vi "Icai 105 - Simultry_9_express.vi"() -> ()   [LabVIEW 2010]
uses:
  <vilib>/Utility/error.llb/DialogType.ctl
  <vilib>/DAQmx/write.llb/DAQmx Write (Analog DBL 1Chan 1Samp).vi
  <vilib>/DAQmx/write.llb/DAQmx Write (Digital 1D Bool 1Chan 1Samp).vi
  <vilib>/DAQmx/write.llb/DAQmx Write (Analog Wfm 1Chan NSamp).vi
  <vilib>/DAQmx/create/channels.llb/DAQmx Create Channel (AO-Voltage-Basic).vi
  <vilib>/daqmx/miscellaneous.llb/DAQmx Fill In Error Info.vi
  <vilib>/Waveform/WDTOps.llb/WDT Append Waveforms DBL.vi
  <vilib>/measure/matone.llb/Extract Single Tone Information 1 Chan.vi
  <vilib>/DAQmx/create/channels.llb/DAQmx Create Channel (DO-Digital Output).vi
  <vilib>/DAQmx/configure/timing.llb/DAQmx Timing (Sample Clock).vi
  <vilib>/measure/NI_MABase.lvlib
  <vilib>/measure/NI_MAPro.lvlib
  Program Files/National Instruments/LabVIEW 2010/resource/objmgr/daqmx.rc
panel:
  in  "rate":dbl=10000000.0
  out "detected frequency 2":dbl format="%.6p"
  out "SampClk.Timebase.Rate":dbl format="%^#_10g"
  in  "Freq Scale Factor":dbl=1.6405228 format="%#_12g"
  out "detected frequency":dbl format="%.6p"
  out "signal out":waveform(dbl)(graph)
  in  "lines":tag="Dev1/port0/line3"
  in  "Rising Logic Output Chan":tag="Dev1/ao2"
  in  "Mod Duration ms":i32=300
  in  "Samples (1Ms/s)":i32=700000
  out "min value":dbl
  in  "Falling Logic Output Chan":tag="Dev1/ao1"
  in  "FM Waveform Channel":tag="Dev1/ao3"
  out "error out":errorcluster caption="error out (DAQ)"
  out "Mod":dbl=118572.0
  out "Numeric 2":dbl=3900000.0 format="%#_7g"
  out "Numeric":dbl=3900000.0 format="%#_7g"
  in  "Pre-Trig Samples":ext=100.0 format="%.2f"
  out "?":dbl=579698.7113293351 format="%#_6f"
  in  "Fs":dbl=1000000.0
  out "#s":dbl=39524.02451426849
  in  "Time int":i32=30000
  in  "Sensitivity":u16(ring)=14 items=["2 nV/fA", "5 nV/fA", "10 nV/fA", "20 nV/fA", "50 nV/fA", "100 nV/fA", "200 nV/fA", "500 nV/fA", "1 uV/pA", "2 uV/pA", "5 uV/pA", "10 uV/pA", "20 uV/pA", "50 uV/pA", "100 uV/pA", "200 uV/pA", "500 uV/pA", "1 mV/nA", "2 mV/nA", "5 mV/nA", "10 mV/nA", "20 mV/nA", "50 mV/nA", "100 mV/nA", "200 mV/nA", "500 mV/nA", "1 V/uA"]
  in  "Detection Bandwidth":u16(ring)=7 items=["10 us/ 25 kHz", "30 us /8.33 kHz", "100 us/ 2.50 kHz", "300 us/ 833 Hz", "1 ms /250 Hz", "3 ms /83.3 Hz", "10 ms/ 25 Hz", "30 ms/ 8.33 Hz", "100 ms/ 2.50 Hz", "300 ms/ 0.833 Hz ", "1 s/ 0.250 Hz", "3 s/ 0.0833 Hz", "10 s/0.025 Hz"]
  in  "SR 830 GPIB Address":i32=8
  in  "Freq 2":dbl=2448.0 format="%_7g"
  out "Iterat #":dbl=10.0
  in  "Iteration":dbl=17.0
  in  "stop 2":bool
  in  "pulse":bool=TRUE
  in  "Start":ext=0.05
  out "?":waveform(dbl)[](graph)
  in  "amplitude 2":dbl=0.25 format="%0.2p"
  in  "?":T1(ring)=enum."Triangle Wave"
  in  "phase 2":dbl format="%.2p"
  in  "Offset 2":dbl=-0.0 format="%#_6p"
  in  "frequency 4":dbl=100.0 format="%0.2p"
  in  "sampling info 4":cluster{"Fs":dbl, "#s":dbl}={"Fs"=1000000.0, "#s"=2500.0} {"Fs" format="%.2p"}
  in  "?":T1(ring)=enum."Triangle Wave"
  in  "offset 4":dbl=-1.0 format="%0.2p"
  in  "phase 4":dbl=90.0 format="%.2p"
  in  "amplitude 4":dbl=1.0 format="%0.2p"
  in  "frequency 1":dbl=100.0 format="%0.2p"
  in  "amplitude 1":dbl=1.0 format="%0.2p"
  in  "sampling info 1":cluster{"Fs":dbl, "#s":dbl}={"Fs"=1000000.0, "#s"=2500.0} {"Fs" format="%.2p"}
  in  "?":T1(ring)=enum."Triangle Wave"
  in  "phase 1":dbl=-90.0 format="%.2p"
  in  "Offset 1":dbl format="%#_6p"
  in  "iterat":dbl
  out "CW":dbl=123571.0
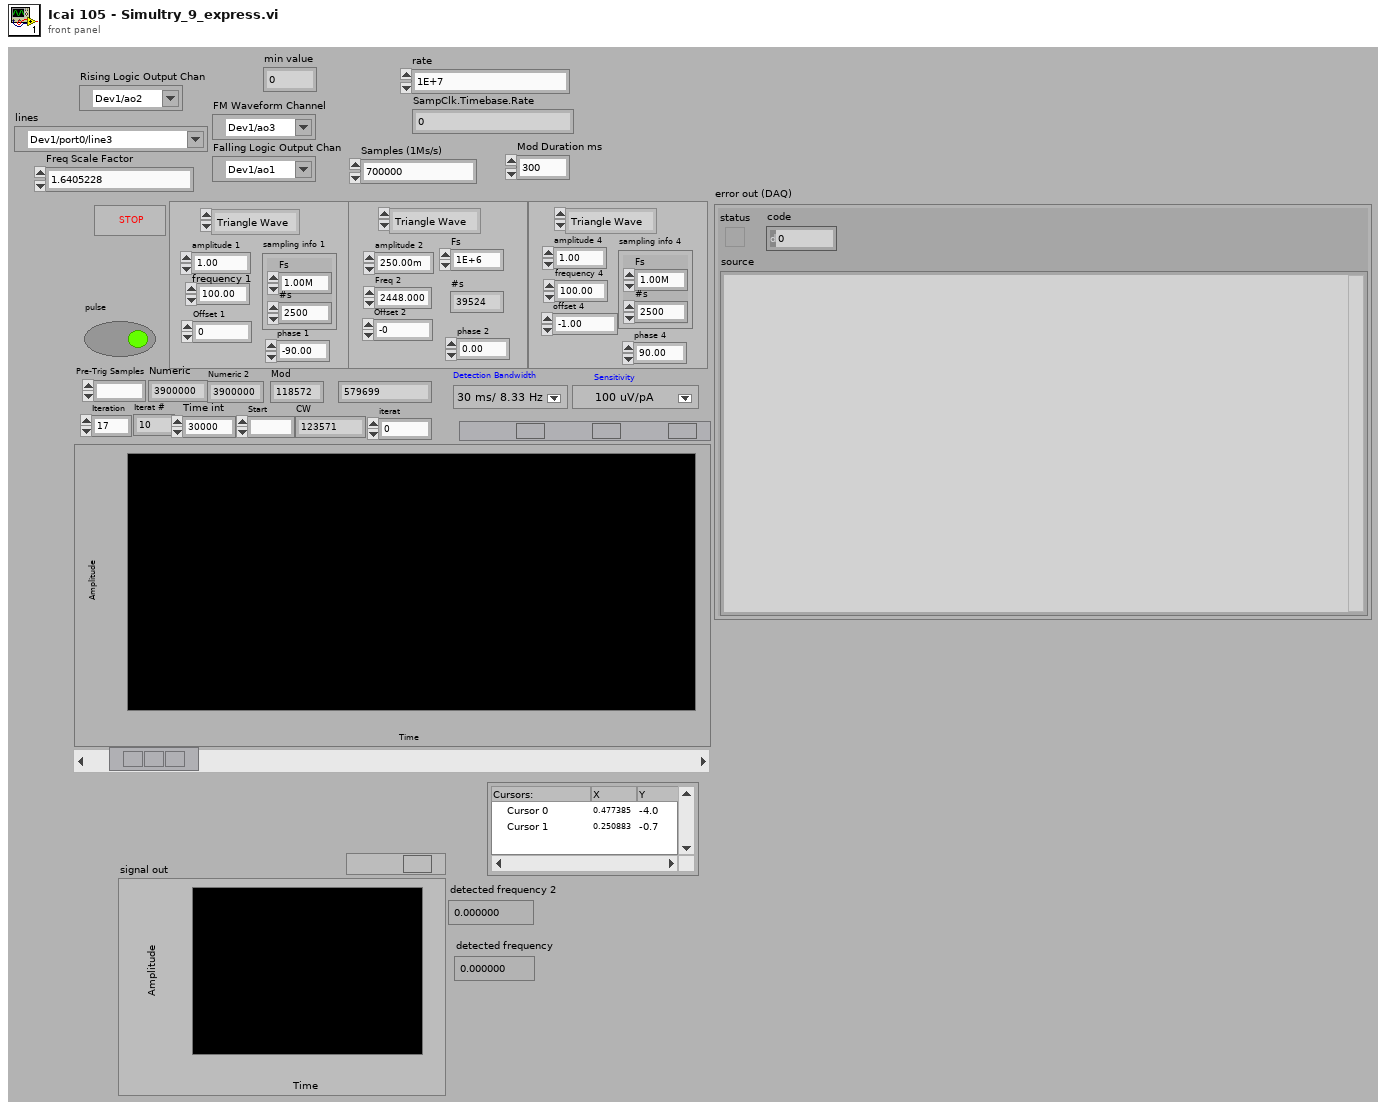
[diagram p1: front panel]
types:
  T1 = enum16{"Sine Wave", "Triangle Wave", "Square Wave", "Sawtooth Wave"}
  T2 = typedef "DialogType.ctl" = u16
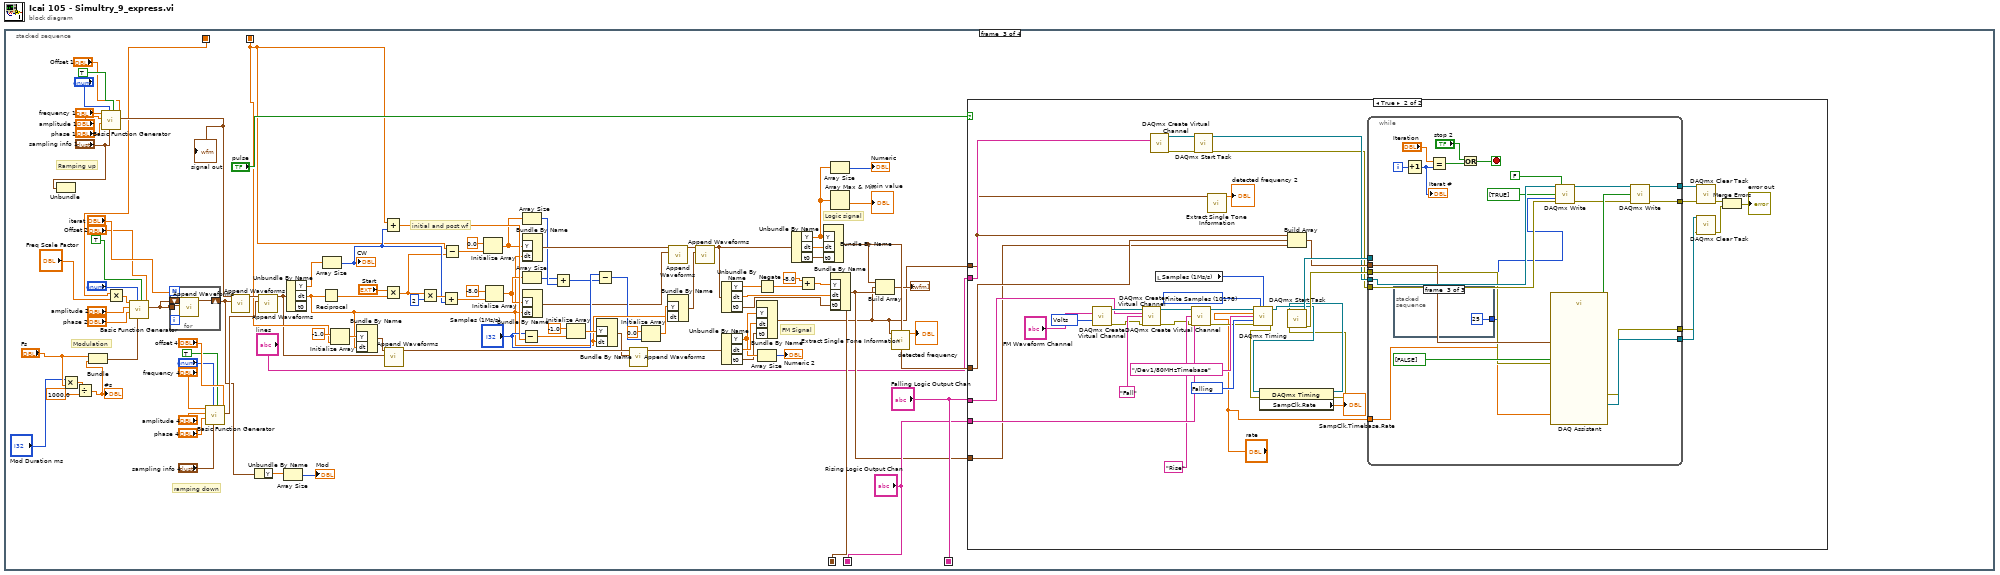
[diagram p0: block diagram]
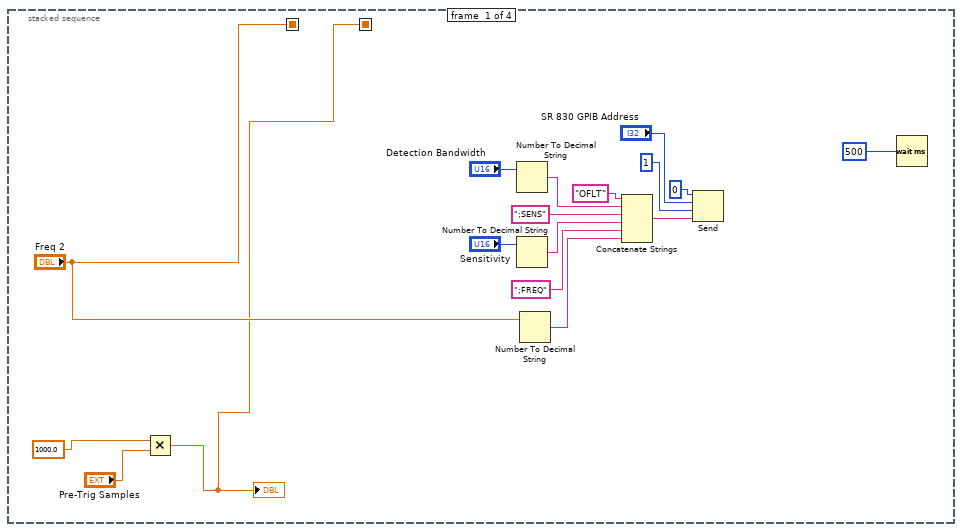
[diagram p2: hidden frame]
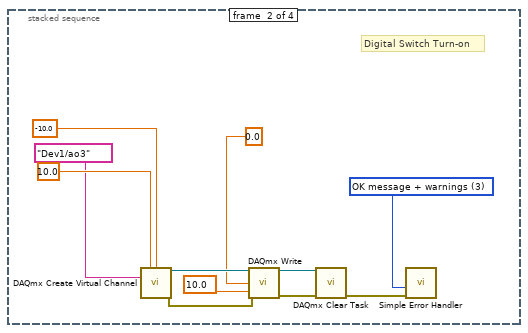
[diagram p3: hidden frame]
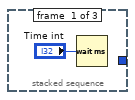
[diagram p5: hidden frame]
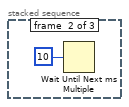
[diagram p6: hidden frame]
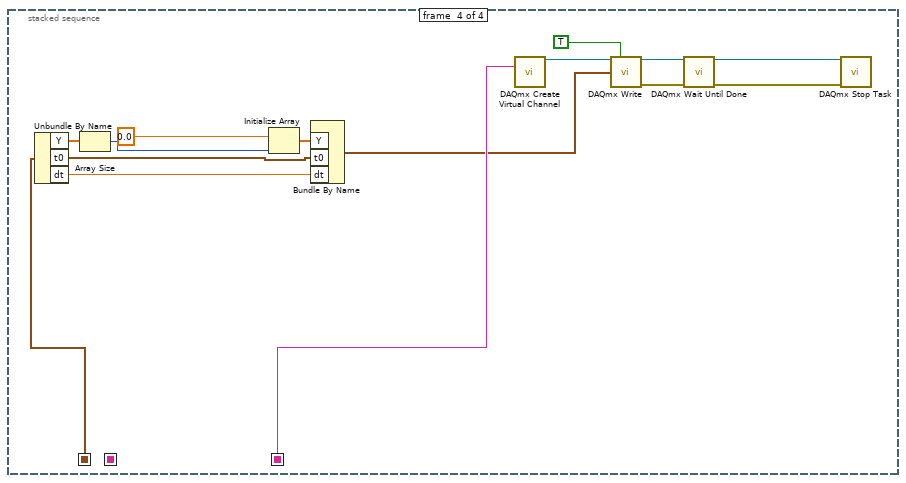
[diagram p7: hidden frame]
diagram:
  n1 = stacked-sequence {
    seq-local: ["Freq 2" _ _ _] -> [_ _ w31 _]
    seq-local: [w1 _ _ _] -> [_ _ w68 _]
    seq-local: [_ _ "Falling Logic Output Chan" _] -> [_ _ _ w196]
    seq-local: [_ _ "Rising Logic Output Chan" _] -> [_ _ _ _]
    seq-local: [_ _ w48 _] -> [_ _ _ w204]
    frame #0 {
      n2 = Multiply(x=1000.0 ("Fs 2"), y="Pre-Trig Samples") -> (x*y=w1:ext)
      "?" <- w1
      n3 = Number To Decimal String(number="Detection Bandwidth") -> (decimal integer string=w16:string)  [unwired: 1 out]
      n4 = Number To Decimal String(number="Sensitivity") -> (decimal integer string=w14:string)  [unwired: 1 out]
      n5 = Number To Decimal String(number="Freq 2") -> (decimal integer string=w5:string)  [unwired: 1 out]
      n6 = Concatenate Strings("OFLT", w16, ";SENS", w14, ";FREQ" ("string"), w5) -> (w13:string)
      n7 = Send(0:0 ("bus"), 2:"SR 830 GPIB Address", 3:i16 1 ("mode"), 5:w13) -> ()  [unwired: 1 in, 3 out]
      n8 = Wait (ms)(milliseconds to wait=500) -> ()  [unwired: 1 out]
    }
    frame #1 {
      w21 = T2 3 items=["no dialog", "OK message", "continue or stop message", "OK message + warnings", "continue/stop + warnings"] ("type of dialog (OK msg:1)")
      # "Digital Switch Turn-on"
      n9 = call-poly <vilib>:"DAQmx Create Virtual Channel.vi"("maximum value"=10.0 ("Maximum Value"), "minimum value"=-10.0 ("Minimum Value"), "physical channels"=tag "Dev1/ao3" ("Physical Channel")) -> ("task out"=w24:refnum<k21>, "error out"=w25:errorcluster)  [unwired: 6 in, 5 out]
      n10 = call-poly <vilib>:"DAQmx Write.vi"("task/channels in"=w24, "data"=0.0 ("Voltage Output"), "timeout"=10.0, "error in"=w25) -> ("task out"=w19:refnum<k21>, "error out"=w20:errorcluster)  [unwired: 1 in, 9 out]
      n11 = call <vilib>:"DAQmx Clear Task.vi"("task in"=w19, "error in"=w20) -> ("error out"=w18:errorcluster)  [unwired: 13 out]
      n12 = call <vilib>:"Simple Error Handler.vi"("type of dialog (OK msg:1)"=w21, "error in (no error)"=w18) -> ()  [unwired: 8 out]
    }
    frame #2 {
      # "initial and post wf"
      # "FM Signal"
      # "Logic signal"
      # "Ramping up"
      # "ramping down"
      # "Modulation"
      n13 = Unbundle("sampling info 1") -> ()  [unwired: 2 out]
      n14 = Multiply(x="Mod Duration ms", y="Fs") -> (x*y=w38:dbl)
      n15 = Divide(x=w38, y=1000.0) -> (x/y=w36:dbl)
      "#s" <- w36
      n16 = Bundle("Fs"="Fs", w36) -> (w72:cluster{"Fs":dbl, dbl})  [unwired: 1 out]
      n17 = call <vilib>:"Basic Function Generator.vi"("offset"="Offset 1", "reset signal"=TRUE, "sampling info"="sampling info 1", "signal type"="?", "phase"="phase 1", "amplitude"="amplitude 1", "frequency"="frequency 1") -> ("signal out"=w106:waveform(dbl))  [unwired: 2 in, 2 out]
      "signal out" <- w106
      n18 = Multiply(x=w31, y="Freq Scale Factor") -> (x*y=w30:dbl)
      n19 = call <vilib>:"Basic Function Generator.vi"("offset"="Offset 2", "reset signal"=TRUE, "sampling info"=w72, "signal type"="?", "phase"="phase 2", "amplitude"="amplitude 2", "frequency"=w30) -> ("signal out"=w34:waveform(dbl))  [unwired: 2 in, 2 out]
      n20 = for {
        N: "iterat" -> [_]
        shift-right: [w194] -> w61
        shift-left: w34 -> [w192]
        tunnel: w34 -> [w193]
        n21 = call-poly <vilib>:"Append Waveforms.vi"("waveform B"=w193, "waveform A"=w192) -> ("waveform out"=w194:waveform(dbl))  [unwired: 1 in, 8 out]
      }
      n22 = call <vilib>:"Basic Function Generator.vi"("offset"="offset 4", "reset signal"=TRUE, "sampling info"="sampling info 4", "signal type"="?", "phase"="phase 4", "amplitude"="amplitude 4", "frequency"="frequency 4") -> ("signal out"=w111:waveform(dbl))  [unwired: 2 in, 2 out]
      n23 = call-poly <vilib>:"Append Waveforms.vi"("waveform B"=w61, "waveform A"=w106) -> ("waveform out"=w105:waveform(dbl))  [unwired: 1 in, 8 out]
      n24 = Unbundle By Name(w61) -> ("Y"=w62:dbl[])
      n25 = call-poly <vilib>:"Append Waveforms.vi"("waveform B"=w111, "waveform A"=w105) -> ("waveform out"=w44:waveform(dbl))  [unwired: 1 in, 8 out]
      n26 = Array Size(array=w62) -> (size(s)=→"Mod":i32)
      n27 = Unbundle By Name(w44) -> ("Y"=w107:dbl[], "dt"=w67:dbl)  [unwired: 1 out]
      n28 = Reciprocal(x=w67) -> (1/x=w69:dbl)
      n29 = Array Size(array=w107) -> (size(s)=w89:i32)
      "CW" <- w89
      n30 = Initialize Array(-1.0 ("DC level"), w68) -> (w96:dbl[])
      n31 = Bundle By Name("Y"=w96, "dt"=w67) -> (w109:waveform(dbl))  [unwired: 1 out]
      n32 = Add(x=w68, y=w89) -> (x+y=w94:ext)
      n33 = Multiply(x="Start", y=w69) -> (x*y=w82:ext)
      n34 = call-poly <vilib>:"Append Waveforms.vi"("waveform B"=w44, "waveform A"=w109) -> ("waveform out"=w110:waveform(dbl))  [unwired: 1 in, 8 out]
      n35 = Multiply(x=w82, y=2) -> (x*y=w90:ext)
      n36 = Add(x=w90, y=w89) -> (x+y=w71:ext)
      n37 = Subtract(x=w68, y=w82) -> (x-y=w83:ext)
      n38 = Initialize Array(0.0 ("Trigger down"), w83) -> (w81:dbl[])
      n39 = Initialize Array(-8.0 ("Trigger up"), w71) -> (w80:dbl[])
      n40 = Subtract(x="Samples (1Ms/s)", y=w94) -> (x-y=w93:ext)
      n41 = Bundle By Name("Y"=w81, "dt"=w67) -> (w85:waveform(dbl))  [unwired: 1 out]
      n42 = Bundle By Name("Y"=w80, "dt"=w67) -> (w42:waveform(dbl))  [unwired: 1 out]
      n43 = Array Size(array=w81) -> (size(s)=w79:i32)
      n44 = Array Size(array=w80) -> (size(s)=w78:i32)
      n45 = Add(x=w78, y=w79) -> (x+y=w77:i32)
      n46 = Initialize Array(-1.0 ("DC level"), w93) -> (w92:dbl[])
      n47 = Subtract(x="Samples (1Ms/s)", y=w77) -> (x-y=w43:i32)
      n48 = Bundle By Name("Y"=w92, "dt"=w67) -> (w91:waveform(dbl))  [unwired: 1 out]
      n49 = call-poly <vilib>:"Append Waveforms.vi"("waveform B"=w91, "waveform A"=w110) -> ("waveform out"=w99:waveform(dbl))  [unwired: 1 in, 8 out]
      n50 = Initialize Array(0.0 ("Trigger down"), w43) -> (w86:dbl[])
      n51 = Bundle By Name("Y"=w86, "dt"=w67) -> (w84:waveform(dbl))  [unwired: 1 out]
      n52 = call-poly <vilib>:"Append Waveforms.vi"("waveform B"=w42, "waveform A"=w85) -> ("waveform out"=w102:waveform(dbl))  [unwired: 1 in, 8 out]
      n53 = call-poly <vilib>:"Append Waveforms.vi"("waveform B"=w84, "waveform A"=w102) -> ("waveform out"=w59:waveform(dbl))  [unwired: 1 in, 8 out]
      n54 = Unbundle By Name(w59) -> ("Y"=w58:dbl[], "dt"=w53:dbl, "t0"=w54:timestamp)
      n55 = Unbundle By Name(w99) -> ("Y"=w64:dbl[], "dt"=w98:dbl, "t0"=w41:timestamp)
      n56 = Bundle By Name("Y"=w64, "dt"=w98, "t0"=w41) -> (w32:waveform(dbl))  [unwired: 1 out]
      n57 = Negate(x=w58) -> (-x=w56:dbl[])
      n58 = Array Size(array=w64) -> (size(s)=→"Numeric 2":i32)
      n59 = Unbundle By Name(w59) -> ("Y"=w60:dbl[], "dt"=w100:dbl, "t0"=w55:timestamp)
      n60 = Add(x=-8.0, y=w56) -> (x+y=w52:dbl[])
      n61 = Bundle By Name("Y"=w60, "dt"=w100, "t0"=w55) -> (w47:waveform(dbl))  [unwired: 1 out]
      n62 = Bundle By Name("Y"=w52, "dt"=w53, "t0"=w54) -> (w48:waveform(dbl))  [unwired: 1 out]
      n63 = Array Size(array=w60) -> (size(s)=→"Numeric":i32)
      n64 = Array Max & Min(array=w60) -> (min value=→"min value":dbl)  [unwired: 3 out]
      n65 = Build Array(w47, w32, w48) -> (→"?":waveform(dbl)[])
      n66 = call-poly <vilib>:"Extract Single Tone Information.vi"("time signal in"=w32) -> ("detected frequency"=→"detected frequency":dbl)  [unwired: 5 in, 5 out]
      n67 = case shown="True" "pulse" {
        tunnel: w32 -> [_ w130]
        tunnel: w47 -> [_ w152]
        tunnel: w48 -> [_ w132]
        tunnel: "Falling Logic Output Chan" -> [_ w165]
        tunnel: "Rising Logic Output Chan" -> [_ w162]
        tunnel: "lines" -> [_ w149]
        frame False {
        }
        frame True {
          w138 = 10348 items=["Volts"=10348, "From Custom Scale"=10065] ("units")
          w157 = 10178 items=["Finite Samples"=10178, "Continuous Samples"=10123, "Hardware Timed Single Point"=12522] ("sample mode")
          w158 = 10171 items=["Rising"=10280, "Falling"=10171] ("active edge")
          n68 = call-poly <vilib>:"DAQmx Create Virtual Channel.vi"("physical channels"="FM Waveform Channel", "units"=w138) -> ("task out"=w166:refnum<k21>, "error out"=w154:errorcluster)  [unwired: 12 in]
          n69 = call-poly <vilib>:"DAQmx Create Virtual Channel.vi"("task in"=w166, "physical channels"=w165, "name to assign"="Fall", "error in"=w154) -> ("task out"=w163:refnum<k21>, "error out"=w155:errorcluster)  [unwired: 10 in]
          n70 = call-poly <vilib>:"DAQmx Create Virtual Channel.vi"("lines"=w149) -> ("task out"=w145:refnum<k21>, "error out"=w139:errorcluster)  [unwired: 13 in]
          n71 = local read "Samples (1Ms/s)"() -> (w146:i32)
          n72 = call-poly <vilib>:"DAQmx Create Virtual Channel.vi"("task in"=w163, "physical channels"=w162, "name to assign"="Rise", "error in"=w155) -> ("task out"=w160:refnum<k21>, "error out"=w156:errorcluster)  [unwired: 10 in]
          n73 = call <vilib>:"DAQmx Start Task.vi"("task/channels in"=w145, "error in"=w139) -> ("task out"=w148:refnum<k21>, "error out"=w147:errorcluster)  [unwired: 12 in]
          n74 = call-poly <vilib>:"Extract Single Tone Information.vi"("time signal in"=w130) -> ("detected frequency"=→"detected frequency 2":dbl)  [unwired: 5 in, 5 out]
          n75 = call-poly <vilib>:"DAQmx Timing.vi"("task/channels in"=w160, "sample mode"=w157, "samples per channel"=w146, "rate"="rate", "source"=tag "/Dev1/80MHzTimebase", "active edge"=w158, "error in"=w156) -> ("task out"=w137:refnum<k21>, "error out"=w134:errorcluster)  [unwired: 7 in]
          n76 = property class="DAQmx Timing"(reference=w137, error in=w134) -> (reference out=w136:refnum<k21>, error out=w135:errorcluster, "SampClk.Rate"=→"SampClk.Timebase.Rate":dbl)
          n77 = call <vilib>:"DAQmx Start Task.vi"("task/channels in"=w136, "error in"=w135) -> ("task out"=w153:refnum<k21>, "error out"=w150:errorcluster)  [unwired: 12 in]
          n78 = Build Array(w130, w152, w132) -> (w151:waveform(dbl)[])
          n79 = while {
            tunnel: w153 -> [_]
            tunnel: w151 -> [w173]
            tunnel: w150 -> [w172]
            tunnel: w148 -> [w182]
            tunnel: w147 -> [w180]
            tunnel: [w175] -> w143
            tunnel: [w174] -> w144
            tunnel: [w171] -> w129
            tunnel: [w170] -> w128
            tunnel: "rate" -> [w169]
            i -> [w185]
            stop <- w186 stop-if-true
            n80 = stacked-sequence {
              tunnel: [_ _ 25 ("timeout (s)")] -> w168
              frame #0 {
                n81 = Wait (ms)(milliseconds to wait="Time int") -> ()  [unwired: 1 out]
              }
              frame #1 {
                n82 = Wait Until Next ms Multiple(millisecond multiple=u32 10) -> ()  [unwired: 1 out]
              }
              frame #2 {
              }
            }
            n83 = Increment(x=w185) -> (x+1=w183:i32)
            "Iterat #" <- w183
            n84 = Equal?(x="Iteration", y=w183) -> (x = y?=w188:bool)
            n85 = Or(x="stop 2", y=w188) -> (x .or. y?=w186:bool)
            n86 = call "DAQ Assistant"("data"=w173, "rate"=w169, "error in"=w172) -> ("task out"=w171:refnum<k21>, "error out"=w170:errorcluster)  [unwired: 15 in]
            n87 = call-poly <vilib>:"DAQmx Write.vi"("task/channels in"=w182, "auto start"=FALSE, "data"=bool[] [TRUE], "timeout"=w168, "error in"=w180) -> ("task out"=w178:refnum<k21>, "error out"=w176:errorcluster)  [unwired: 8 in, 1 out]
            n88 = call-poly <vilib>:"DAQmx Write.vi"("task/channels in"=w178, "data"=bool[] [FALSE], "error in"=w176) -> ("task out"=w174:refnum<k21>, "error out"=w175:errorcluster)  [unwired: 10 in, 1 out]
          }
          n89 = call <vilib>:"DAQmx Clear Task.vi"("task in"=w144, "error in"=w143) -> ("error out"=w142:errorcluster)  [unwired: 13 in]
          n90 = call <vilib>:"DAQmx Clear Task.vi"("task in"=w129, "error in"=w128) -> ("error out"=w140:errorcluster)  [unwired: 13 in]
          n91 = Merge Errors(w142, w140) -> (→"error out":errorcluster)
        }
      }
    }
    frame #3 {
      n92 = Unbundle By Name(w204) -> ("Y"=w201:dbl[], "t0"=w203:timestamp, "dt"=w202:dbl)
      n93 = Array Size(array=w201) -> (size(s)=w200:i32)
      n94 = Initialize Array(0.0 ("element"), w200) -> (w198:dbl[])
      n95 = Bundle By Name("Y"=w198, "t0"=w203, "dt"=w202) -> (w195:waveform(dbl))  [unwired: 1 in]
      n96 = call-poly <vilib>:"DAQmx Create Virtual Channel.vi"("physical channels"=w196) -> ("task out"=w197:refnum<k21>)  [unwired: 13 in, 1 out]
      n97 = call-poly <vilib>:"DAQmx Write.vi"("task/channels in"=w197, "auto start"=TRUE, "data"=w195) -> ("task out"=w205:refnum<k21>, "error out"=w208:errorcluster)  [unwired: 10 in, 1 out]
      n98 = call <vilib>:"DAQmx Wait Until Done.vi"("task/channels in"=w205, "error in"=w208) -> ("task out"=w207:refnum<k21>, "error out"=w209:errorcluster)  [unwired: 12 in]
      n99 = call <vilib>:"DAQmx Stop Task.vi"("task/channels in"=w207, "error in"=w209) -> ()  [unwired: 12 in, 2 out]
    }
  }
